vi "z-split sum difference.vi"(6 "split type":u16(ring) items=["Horizontal", "Vertical"], 10 "G input":dbl[][](array[numeric]), 11 "center":dbl) -> (1 "left/top":dbl[][](graph), 2 "right/bottom":dbl[][](graph), 3 "difference":dbl)   [LabVIEW 2015]
doc: "This vi splits the input image horizontally or vertically into subimages and finds the difference between the sum of elements in each part. Additionally, the subimages are returned with padded zeros to match the size of the input image. For z-value measurement the x,y position should be inside the image region\n\nINPUT\ncenter - x or y position of the particle\nG input - local gradient image\nsplit type - horizontal or vertical.\n\nOUTPUT\ndifferense - difference between sums of opposite halves of input image\nrigth/bottom, left/top - splitted image padded with zeros to match the input image size\n\nAuthor: Anatolii Kashchuk"
panel:
  # "Author: Anatolii Kashchuk"
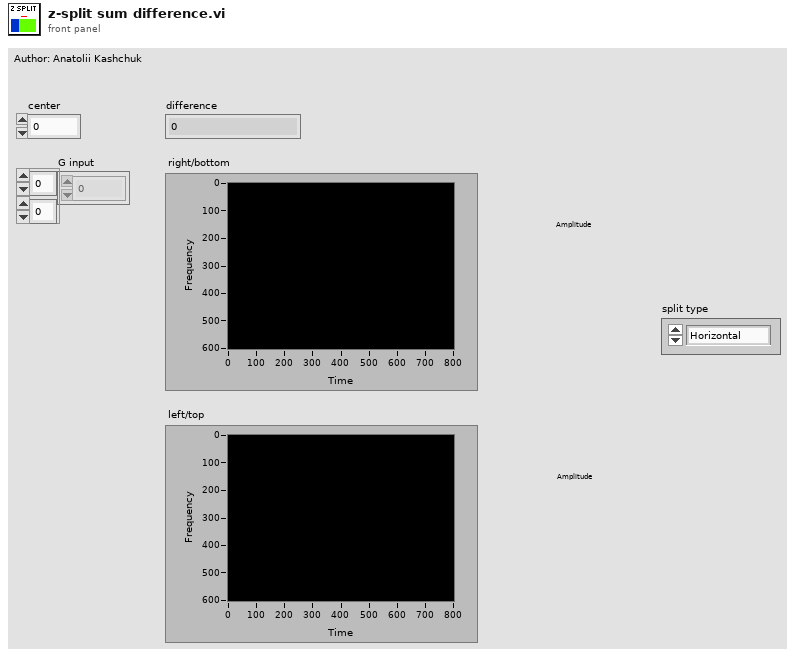
[diagram p1: front panel]
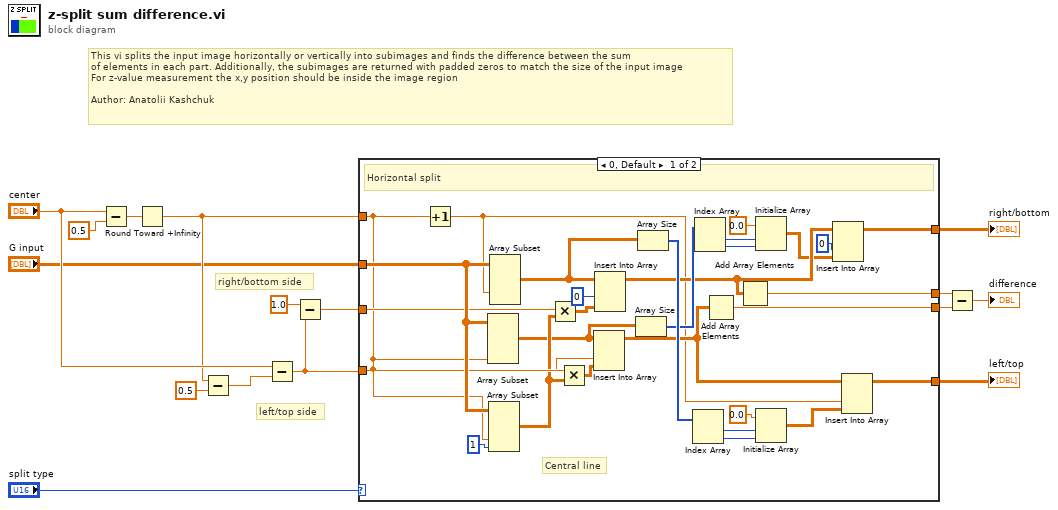
[diagram p0: block diagram]
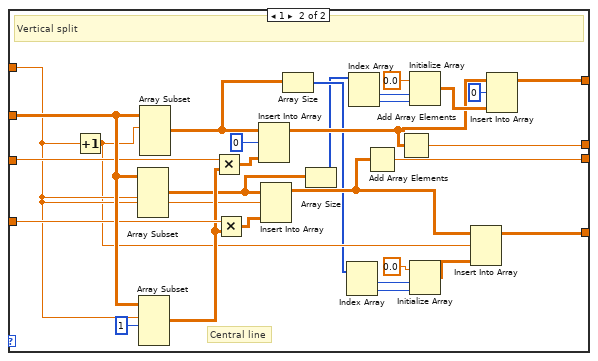
[diagram p2: hidden frame]
diagram:
  # "This vi splits the input image horizontally or vertically into subimages and finds the difference between the sum \nof elements in each part. Additionally, the subimages are returned with padded zeros to match the size of the input image\nFor z-value measurement the x,y position should be inside the image region\n\nAuthor: Anatolii Kashchuk"
  # "left/top side"
  # "right/bottom side"
  n1 = Subtract(x="center", y=0.5) -> (x-y=w11:dbl)
  n2 = Round Toward +Infinity(x=w11) -> (ceil(x): smallest int >= x=w10:dbl)
  n3 = Subtract(x=w10, y=0.5) -> (x-y=w8:dbl)
  n4 = Subtract(x="center", y=w8) -> (x-y=w6:dbl)
  n5 = Subtract(x=1.0, y=w6) -> (x-y=w5:dbl)
  n6 = case shown="0, Default" "split type" {
    tunnel: "G input" -> [w44 w74]
    tunnel: [w31 w56] -> w2
    tunnel: [w20 w46] -> w1
    tunnel: w10 -> [w26 w66]
    tunnel: w6 -> [w42 w68]
    tunnel: w5 -> [w39 w69]
    tunnel: [w28 w62] -> w3
    tunnel: [w27 w63] -> w4
    frame 0, Default {
      # "Central line"
      # "Horizontal split"
      n7 = Increment(x=w26) -> (x+1=w19:dbl)
      n8 = Array Subset(array=w44, length (col)=w26) -> (w36:dbl[][])  [unwired: 3 in]
      n9 = Array Subset(array=w44, index (col)=w26, length (col)=1 ("length")) -> (w40:dbl[][])  [unwired: 2 in]
      n10 = Array Subset(array=w44, index (col)=w19) -> (w37:dbl[][])  [unwired: 3 in]
      n11 = Multiply(x=w39, y=w40) -> (x*y=w41:dbl[][])
      n12 = Multiply(x=w42, y=w40) -> (x*y=w43:dbl[][])
      n13 = Insert Into Array(array=w36, index (col)=w26, new element=w43) -> (w29:dbl[][])  [unwired: 1 in]
      n14 = Insert Into Array(array=w37, index (col)=0 ("disabled index (col)"), new element=w41) -> (w21:dbl[][])  [unwired: 1 in]
      n15 = Array Size(array=w36) -> (size(s)=w22:i32[])
      n16 = Array Size(array=w37) -> (size(s)=w32:i32[])
      n17 = Index Array(array=w32) -> (element #1=w34:i32, element #2=w35:i32)  [unwired: 2 in]
      n18 = Index Array(array=w22) -> (element #1=w24:i32, element #2=w25:i32)  [unwired: 2 in]
      n19 = Add Array Elements(numeric array=w29) -> (sum=w28:dbl)
      n20 = Add Array Elements(numeric array=w21) -> (sum=w27:dbl)
      n21 = Initialize Array(0.0 ("element"), w24, w25) -> (w17:dbl[][])
      n22 = Initialize Array(0.0 ("element"), w34, w35) -> (w30:dbl[][])
      n23 = Insert Into Array(array=w21, index (col)=0 ("disabled index (col)"), new element=w17) -> (w20:dbl[][])  [unwired: 1 in]
      n24 = Insert Into Array(array=w29, index (col)=w19, new element=w30) -> (w31:dbl[][])  [unwired: 1 in]
    }
    frame 1 {
      # "Central line"
      # "Vertical split"
      n25 = Increment(x=w66) -> (x+1=w55:dbl)
      n26 = Array Subset(array=w74, length (row)=w66) -> (w64:dbl[][])  [unwired: 3 in]
      n27 = Array Subset(array=w74, index (row)=w66, length (row)=1 ("length")) -> (w67:dbl[][])  [unwired: 2 in]
      n28 = Array Subset(array=w74, index (row)=w55) -> (w65:dbl[][])  [unwired: 3 in]
      n29 = Multiply(x=w69, y=w67) -> (x*y=w72:dbl[][])
      n30 = Multiply(x=w68, y=w67) -> (x*y=w71:dbl[][])
      n31 = Insert Into Array(array=w65, index (row)=0 ("disabled index (col)"), new element=w72) -> (w50:dbl[][])  [unwired: 1 in]
      n32 = Insert Into Array(array=w64, index (row)=w66, new element=w71) -> (w57:dbl[][])  [unwired: 1 in]
      n33 = Array Size(array=w65) -> (size(s)=w49:i32[])
      n34 = Array Size(array=w64) -> (size(s)=w48:i32[])
      n35 = Index Array(array=w49) -> (element #1=w60:i32, element #2=w61:i32)  [unwired: 2 in]
      n36 = Index Array(array=w48) -> (element #1=w53:i32, element #2=w54:i32)  [unwired: 2 in]
      n37 = Add Array Elements(numeric array=w57) -> (sum=w62:dbl)
      n38 = Add Array Elements(numeric array=w50) -> (sum=w63:dbl)
      n39 = Initialize Array(0.0 ("element"), w53, w54) -> (w51:dbl[][])
      n40 = Initialize Array(0.0 ("element"), w60, w61) -> (w58:dbl[][])
      n41 = Insert Into Array(array=w57, index (row)=w55, new element=w58) -> (w56:dbl[][])  [unwired: 1 in]
      n42 = Insert Into Array(array=w50, index (row)=0 ("disabled index (col)"), new element=w51) -> (w46:dbl[][])  [unwired: 1 in]
    }
  }
  "right/bottom" <- w1
  "left/top" <- w2
  n43 = Subtract(x=w4, y=w3) -> (x-y=→"difference":dbl)
